vi "Group_OpenWfms.vi"(8 "error in (no error)":errorcluster, 11 "Group in":refnum<class "Group.lvclass">) -> (0 "error out":errorcluster, 3 "Group out":refnum<class "Group.lvclass">)   [LabVIEW 2023, in "Group.lvclass"]
doc: "Mid level VI that triggers each Wfm channel to open their Waveform session reference for use in the VeriStand Engine during execution."
uses:
  Group.lvclass
  Group.lvclass/Group.ctl
  Channel/Channel.lvclass
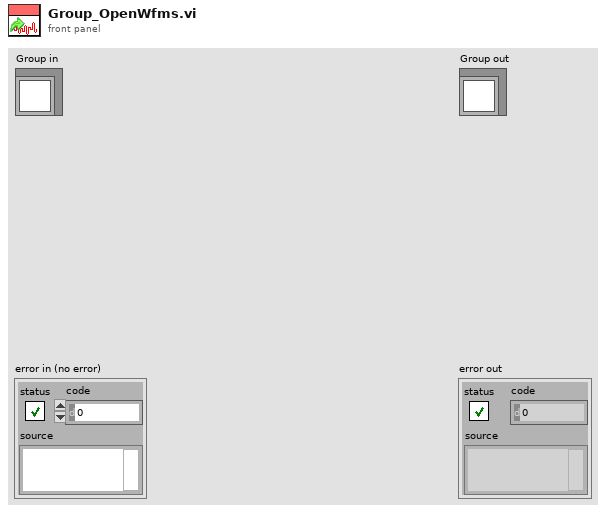
[diagram p1: front panel]
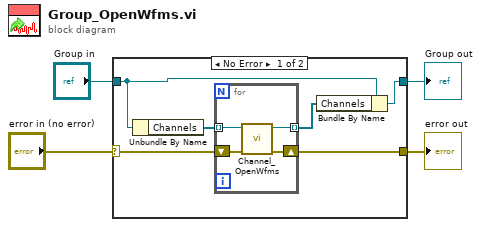
[diagram p0: block diagram]
diagram:
  n1 = case shown="No Error" "error in (no error)" {
    selector: "error in (no error)" -> [w8 w16]
    tunnel: [w7 w16] -> w3
    tunnel: [w9 w15] -> w1
    tunnel: "Group in" -> [w10 w15]
    frame No Error {
      n2 = Unbundle By Name(w10) -> ("Channels"=w6:refnum<class "Channel.lvclass">[])
      n3 = for {
        shift-right: [w12] -> w7
        shift-left: w8 -> [w11]
        tunnel: w6 -> [w14] mode=indexing
        tunnel: [w13] -> w5 mode=indexing
        n4 = call-dynamic "Channel_OpenWfms.vi"("error in (no error)"=w11, "Channel in"=w14) -> ("error out"=w12:errorcluster, "Channel out"=w13:refnum<class "Channel.lvclass">)  [unwired: 8 in]
      }
      n5 = Bundle By Name(cluster=w10, "Channels"=w5) -> (w9:refnum<class "Group.lvclass">)
    }
    frame Error {
    }
  }
  "error out" <- w3
  "Group out" <- w1
